vi "RM-config-motion.vi"(6 "Dec":dbl, 7 "Band":dbl, 8 "error in (no error)":errorcluster, 9 "Acc":dbl, 10 "speed":dbl, 11 "MB_Master_Serial输入":refnum<class "MB_Master_Serial.lvclass">) -> (0 "error out":errorcluster, 3 "MB_Master_Serial输出":refnum<class "MB_Master_Serial.lvclass">)   [LabVIEW 2014]
uses:
  <vilib>/Plasmionique/MB Master/MB_Master_Serial/MB_Master_Serial.lvclass
  <vilib>/Plasmionique/MB Master/MB Master.lvlib
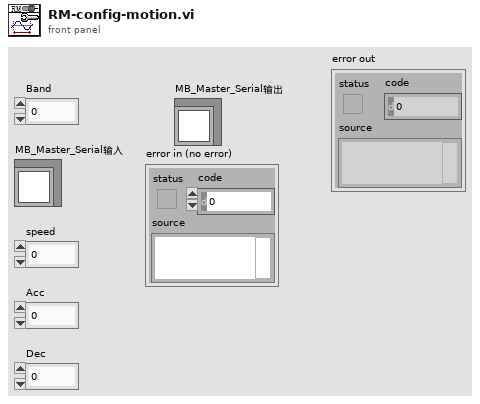
[diagram p1: front panel]
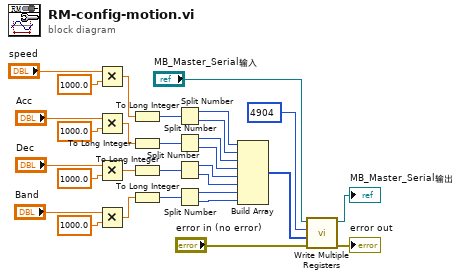
[diagram p0: block diagram]
diagram:
  n1 = Multiply(x="speed", y=1000.0) -> (x*y=w14:dbl)
  n2 = Multiply(x="Acc", y=1000.0) -> (x*y=w18:dbl)
  n3 = Multiply(x="Dec", y=1000.0) -> (x*y=w21:dbl)
  n4 = Multiply(x="Band", y=1000.0) -> (x*y=w26:dbl)
  n5 = To Long Integer(number=w14) -> (32bit integer=w15:i32)
  n6 = To Long Integer(number=w18) -> (32bit integer=w22:i32)
  n7 = To Long Integer(number=w21) -> (32bit integer=w23:i32)
  n8 = To Long Integer(number=w26) -> (32bit integer=w27:i32)
  n9 = Split Number(x=w15) -> (hi(x)=w4:u16, lo(x)=w5:u16)
  n10 = Split Number(x=w22) -> (hi(x)=w6:u16, lo(x)=w7:u16)
  n11 = Split Number(x=w23) -> (hi(x)=w8:u16, lo(x)=w9:u16)
  n12 = Split Number(x=w27) -> (hi(x)=w10:u16, lo(x)=w11:u16)
  n13 = Build Array(w4, w5, w6, w7, w8, w9, w10, w11) -> (w28:u16[])
  n14 = call <vilib>:"Write Multiple Registers.vi"("error in (no error)"="error in (no error)", "values"=w28, "starting address"=u16 4904, "MB session in"="MB_Master_Serial输入") -> ("error out"=→"error out":errorcluster, "MB session out"=→"MB_Master_Serial输出":refnum<class "MB_Master_Serial.lvclass">)  [unwired: 6 in]
